vi "AlarmQueryActiveTrendInstancesResponse_Parse.vi"(8 "error in (no error)":errorcluster, 11 "Message":T8) -> (0 "error out":errorcluster, 1 "Body":T1, 2 "Header":T6, 3 "AlarmQueryActiveTrendInstancesResponse":T5)   [LabVIEW 2017]
uses:
  <vilib>/addons/InsightCM/MessageBus/Base/controls/Message.ctl
  <vilib>/addons/InsightCM/MessageBus/Base/controls/MessageHeader.ctl
  <vilib>/addons/InsightCM/MessageBus/Base/controls/KeyValuePair.ctl
  <vilib>/addons/InsightCM/MessageBus/MessageLibrary/TrendAlarm/controls/AlarmQueryActiveTrendInstancesResponse.ctl
  <vilib>/addons/InsightCM/MessageBus/MessageLibrary/TrendAlarm/controls/AlarmQueryActiveTrendInstancesResponseBody.ctl
  <vilib>/addons/InsightCM/MessageBus/Base/controls/TrendAlarmInstance.ctl
  <vilib>/addons/InsightCM/MessageBus/Base/controls/TrendAlarmTransition.ctl
  <vilib>/addons/InsightCM/MessageBus/Base/controls/Annotation.ctl
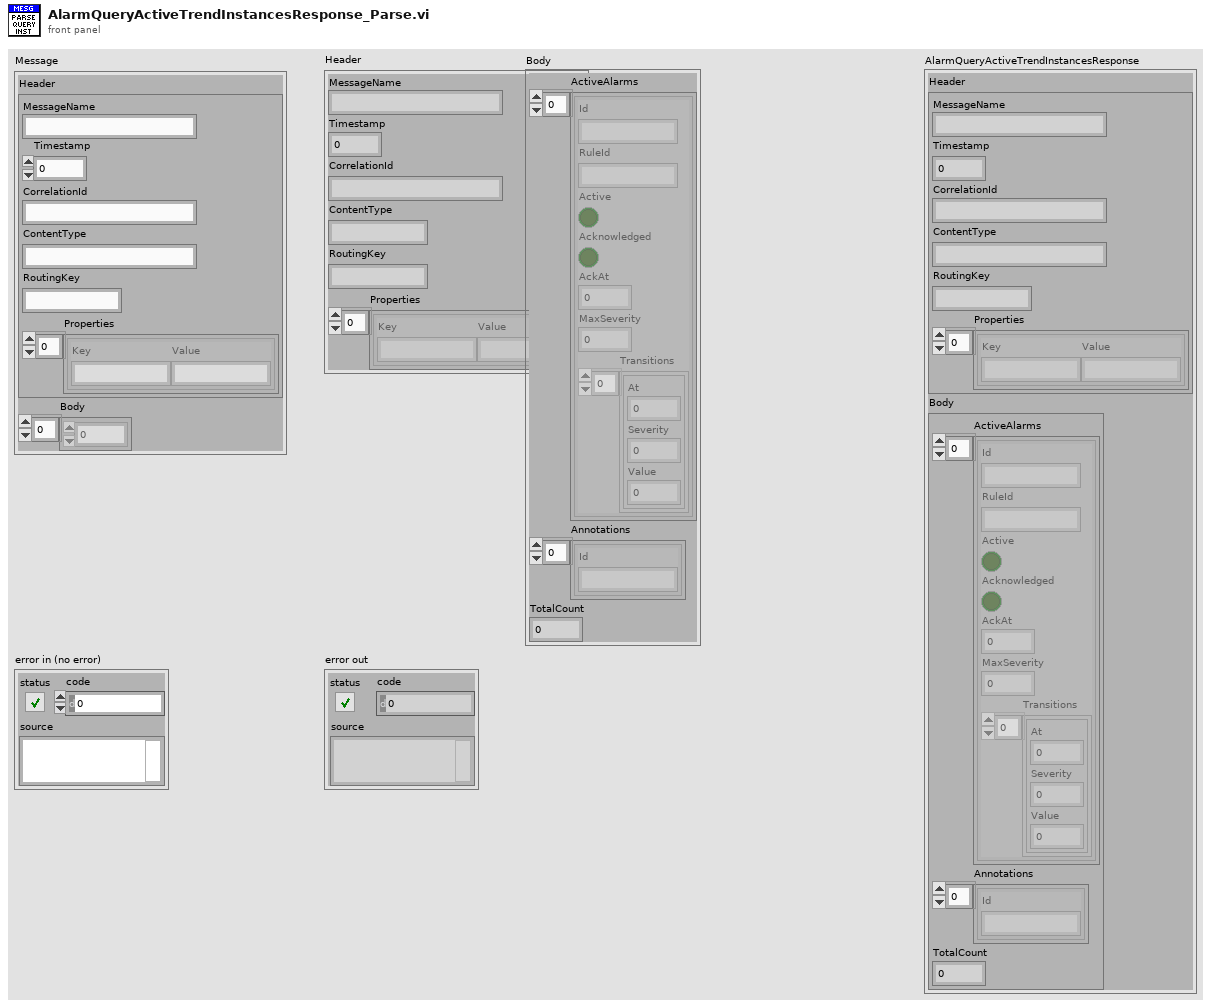
[diagram p1: front panel]
types:
  T1 = typedef "AlarmQueryActiveTrendInstancesResponseBody.ctl" = cluster{"ActiveAlarms":T2[], "Annotations":T4[], "TotalCount":i32}
  T2 = typedef "TrendAlarmInstance.ctl" = cluster{"Id":string, "RuleId":string, "Active":bool, "Acknowledged":bool, "AckAt":i64, "MaxSeverity":i32, "Transitions":T3[]}
  T3 = typedef "TrendAlarmTransition.ctl" = cluster{"At":i64, "Severity":i32, "Value":dbl}
  T4 = typedef "Annotation.ctl" = cluster{"Id":string}
  T5 = typedef "AlarmQueryActiveTrendInstancesResponse.ctl" = cluster{"Header":T6, "Body":T1}
  T6 = typedef "MessageHeader.ctl" = cluster{"MessageName":string, "Timestamp":i64, "CorrelationId":string, "ContentType":string, "RoutingKey":string, "Properties":T7[]}
  T7 = typedef "KeyValuePair.ctl" = cluster{"Key":string, "Value":string}
  T8 = typedef "Message.ctl" = cluster{"Header":T6, "Body":u8[]}
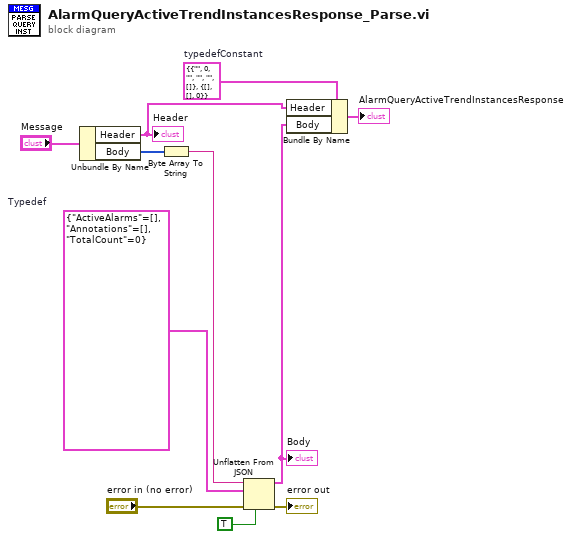
[diagram p0: block diagram]
diagram:
  w3 = T5 {"Header"={"MessageName"="", "Timestamp"=0, "CorrelationId"="", "ContentType"="", "RoutingKey"="", "Properties"=[]}, "Body"={"ActiveAlarms"=[], "Annotations"=[], "TotalCount"=0}}  # typedefConstant
  w7 = T1 {"ActiveAlarms"=[], "Annotations"=[], "TotalCount"=0}  # Typedef
  n1 = Unbundle By Name("Message") -> ("Header"=w9:T6, "Body"=w1:u8[])
  "Header" <- w9
  n2 = Byte Array To String(unsigned byte array=w1) -> (string=w6:string)
  n3 = Unflatten From JSON(JSON string=w6, type and defaults=w7, default null elements? (F)=TRUE, error in (no error)="error in (no error)") -> (value=w5:T1, error out=→"error out":errorcluster)  [unwired: 3 in]
  "Body" <- w5
  n4 = Bundle By Name(cluster=w3, "Header"=w9, "Body"=w5) -> (→"AlarmQueryActiveTrendInstancesResponse":T5)
